vi "Sensor HW Drive Read.vi"(8 "Error":errorcluster, 10 "Config HW Drive Values":T1={"System Ver"=0, "Auto Angle PID"={"Gains"={"P"=0.1, "I"=0.0, "D"=0.0, "F"=0.0}, "Error Allowed"={"High"=0.0, "Low"=0.0}, "I Zone"={"High"=0.0, "Low"=0.0}, "Peak Out 0-1"={"High"=0.0, "Low"=0.0}, "Max I Accu"={"High"=0.0, "Low"=0.0}}, "Frame"={"Length"=33.0, "Width"=0.0}, "Drive Data"={"CPR"=14.0, "RevMotor/Wheel"=6.67, "Wheel Diameter (in)"=4.0}, "Speed Full Scale"=5000.0, "Steer Data"={"CPR"=1024.0}} {"Auto Angle PID"."Max I Accu"."Low" format="%#.8f"; "Auto Angle PID"."Max I Accu"."High" format="%#.8f"; "Auto Angle PID"."Gains"."F" format="%#.8f"; "Auto Angle PID"."Gains"."D" format="%#.8f"; "Auto Angle PID"."Gains"."I" format="%#.8f"; "Auto Angle PID"."Gains"."P" format="%#.8f"; "Auto Angle PID"."Error Allowed"."Low" format="%#.8f"; "Auto Angle PID"."Error Allowed"."High" format="%#.8f"; "Auto Angle PID"."I Zone"."Low" format="%#.8f"; "Auto Angle PID"."I Zone"."High" format="%#.8f"; "Auto Angle PID"."Peak Out 0-1"."Low" format="%#.8f"; "Auto Angle PID"."Peak Out 0-1"."High" format="%#.8f"}, 11 "Drive Ref":T8[](array[typedef])) -> (0 "Error Out":errorcluster, 2 "Drive Velocities (0-1) Out":dbl[](array[numeric]), 3 "Drive Refs Out":T8[](array[typedef]), 5 "Drive Positions (Rev) Out":dbl[](array[numeric]))   [LabVIEW 2023, in "Swerve-SteerSRX-DriveSpark-AbsAnalog_ACT.lvlib"]
uses:
  Swerve-SteerSRX-DriveSpark-AbsAnalog_ACT.lvlib
  <vilib>/Rock Robotics/WPI/MotorControl/WPI_MotorControlDeviceRef.ctl
  <vilib>/Rock Robotics/WPI/MotorControl/WPI_MotorControlType.ctl
  <vilib>/Rock Robotics/SystemInterfaces/DIO/FPGA_DIOPWMChannel.ctl
  <vilib>/Rock Robotics/WPI/PWM/WPI_PWMDeadband.ctl
  <vilib>/Rock Robotics/SystemInterfaces/DIO/FPGA_DIOChannel.ctl
  Cluster_System Config_Values.ctl
  Shared Code/TypeDefs/Cluster_SW PID Config.ctl
  Shared Code/TypeDefs/Cluster_PID Gains.ctl
  Shared Code/TypeDefs/Cluster_High-Low.ctl
  Type Defs/Cluster_Length and Width.ctl
  Shared Code/TypeDefs/Cluster_Config_Swerve_Drive Param.ctl
  Shared Code/TypeDefs/Cluster_Config_Swerve_Steer Parm.ctl
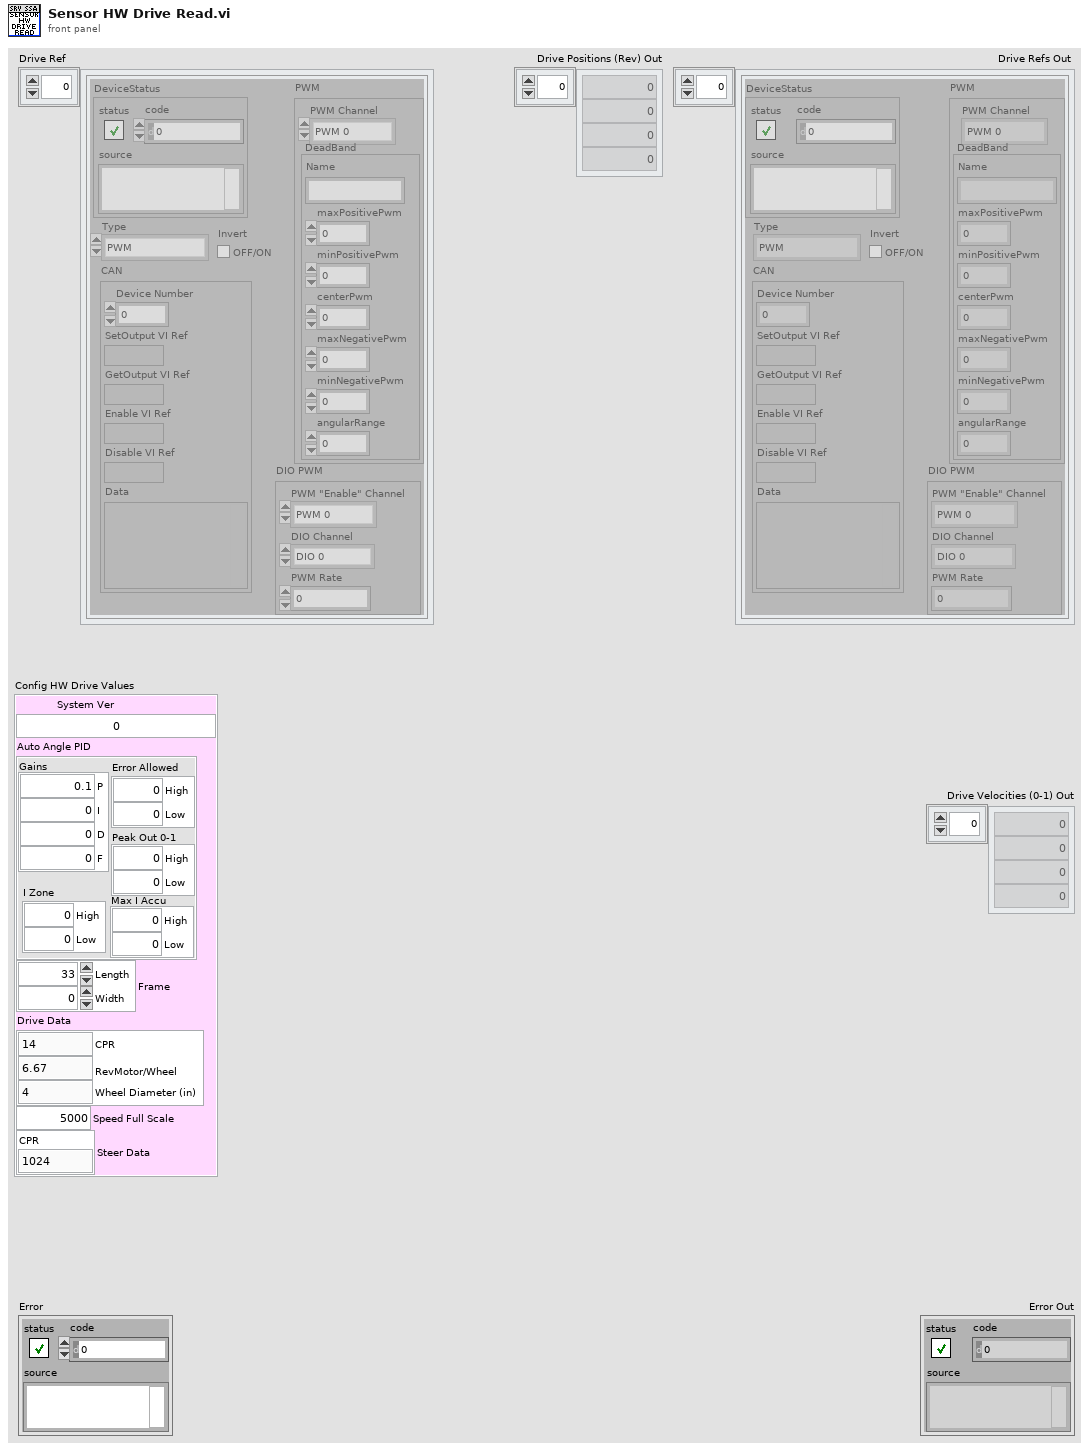
[diagram p1: front panel]
types:
  T1 = typedef "Swerve-SteerSRX-DriveSpark-AbsAnalog_ACT.lvlib/Cluster_System Config_Values.ctl" = cluster{"System Ver":u64, "Auto Angle PID":T2, "Frame":T5, "Drive Data":T6, "Speed Full Scale":dbl, "Steer Data":T7}
  T2 = typedef "Cluster_SW PID Config.ctl" = cluster{"Gains":T3, "Error Allowed":T4, "I Zone":T4, "Peak Out 0-1":T4, "Max I Accu":T4}
  T3 = typedef "Cluster_PID Gains.ctl" = cluster{"P":dbl, "I":dbl, "D":dbl, "F":dbl}
  T4 = typedef "Cluster_High-Low.ctl" = cluster{"High":dbl, "Low":dbl}
  T5 = typedef "Cluster_Length and Width.ctl" = cluster{"Length":dbl, "Width":dbl}
  T6 = typedef "Cluster_Config_Swerve_Drive Param.ctl" = cluster{"CPR":dbl, "RevMotor/Wheel":dbl, "Wheel Diameter (in)":dbl}
  T7 = typedef "Cluster_Config_Swerve_Steer Parm.ctl" = cluster{"CPR":dbl}
  T8 = typedef "WPI_MotorControlDeviceRef.ctl" = cluster{"DeviceStatus":errorcluster, "Type":T9, "PWM":cluster{"PWM Channel":T10, "DeadBand":T11}, "CAN":cluster{"Device Number":u8, "SetOutput VI Ref":variant, "GetOutput VI Ref":variant, "Enable VI Ref":variant, "Disable VI Ref":variant, "Data":variant}, "Invert":bool, "DIO PWM":cluster{"PWM \"Enable\" Channel":T10, "DIOChannel":T12, "PWM Rate":dbl}}
  T9 = typedef "WPI_MotorControlType.ctl" = enum16{"PWM", "CAN", "DIO PWM"}
  T10 = typedef "FPGA_DIOPWMChannel.ctl" = enum8{"PWM 0", "PWM 1", "PWM 2", "PWM 3", "PWM 4", "PWM 5", "PWM 6", "PWM 7", "PWM 8", "PWM 9", "PWM MXP 0", "PWM MXP 1", "PWM MXP 2", "PWM MXP 3", "PWM MXP 4", "PWM MXP 5", "PWM MXP 6", "PWM MXP 7", "PWM MXP 8", "PWM MXP 9", "Invalid"}
  T11 = typedef "WPI_PWMDeadband.ctl" = cluster{"Name":string, "maxPositivePwm":i32, "minPositivePwm":i32, "centerPwm":i32, "maxNegativePwm":i32, "minNegativePwm":i32, "angularRange":u16}
  T12 = typedef "FPGA_DIOChannel.ctl" = enum8{"DIO 0", "DIO 1", "DIO 2", "DIO 3", "DIO 4", "DIO 5", "DIO 6", "DIO 7", "DIO 8", "DIO 9", "DIO MXP 0", "DIO MXP 1", "DIO MXP 2", "DIO MXP 3", "DIO MXP 4", "DIO MXP 5", "DIO MXP 6", "DIO MXP 7", "DIO MXP 8", "DIO MXP 9", "DIO MXP 10", "DIO MXP 11", "DIO MXP 12", "DIO MXP 13", "DIO MXP 14", "DIO MXP 15", "SPI Port CS1", "SPI Port CS2", "SPI Port CS3", "SPI Port MISO", "SPI Port MOSI", "Invalid"}
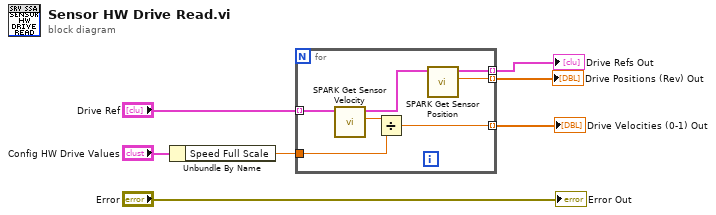
[diagram p0: block diagram]
diagram:
  n1 = Unbundle By Name("Config HW Drive Values") -> ("Speed Full Scale"=w5:dbl)
  n2 = for {
    tunnel: "Drive Ref" -> [w12] mode=indexing
    tunnel: w5 -> [w14]
    tunnel: [w13] -> w4 mode=indexing
    tunnel: [w9] -> w3 mode=indexing
    tunnel: [w8] -> w1 mode=indexing
    n3 = call <vilib>:"SPARK Get Sensor Velocity.vi"("MotorControlDevRef in"=w12) -> ("Sensor Velocity"=w10:dbl, "MotorControlDevRef out"=w11:T8)  [unwired: 7 in, 2 out]
    n4 = Divide(x=w10, y=w14) -> (x/y=w13:dbl)
    n5 = call <vilib>:"SPARK Get Sensor Position.vi"("MotorControlDevRef in"=w11) -> ("Sensor Position"=w9:dbl, "MotorControlDevRef out"=w8:T8)  [unwired: 7 in, 2 out]
  }
  "Drive Refs Out" <- w1
  "Drive Velocities (0-1) Out" <- w4
  "Drive Positions (Rev) Out" <- w3
  "Error Out" <- "Error"
